vi "2일차2.vi"() -> ()   [LabVIEW 2014]
panel:
  in  "정지":bool=TRUE
  out "웨이브폼 차트":dbl(graph)
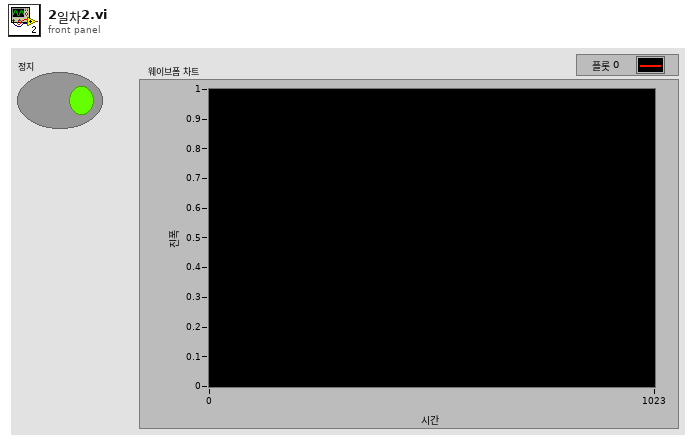
[diagram p1: front panel]
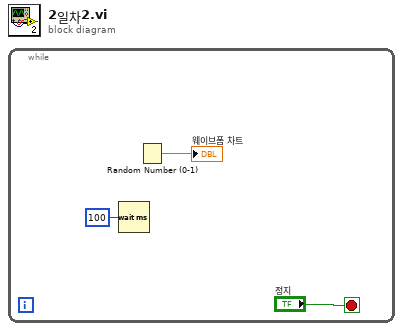
[diagram p0: block diagram]
diagram:
  n1 = while {
    stop <- "정지" stop-if-true
    n2 = Wait (ms)(milliseconds to wait=u32 100 ("대기 시간(ms)")) -> ()  [unwired: 1 out]
    n3 = Random Number (0-1)() -> (number: 0 to 1=→"웨이브폼 차트":dbl)
  }
